vi "get Test by id.vi"(8 "error in (no error)":errorcluster, 10 "id":i32, 11 "Norm in":refnum<class "Norm.lvclass">) -> (0 "error out":errorcluster, 2 "Test.lvclass":refnum<class "Test.lvclass">, 3 "Norm out":refnum<class "Norm.lvclass">)   [LabVIEW 2013, in "DatenKlassen.lvlib" / "Norm.lvclass"]
uses:
  Norm.lvclass
  Test/Test.lvclass
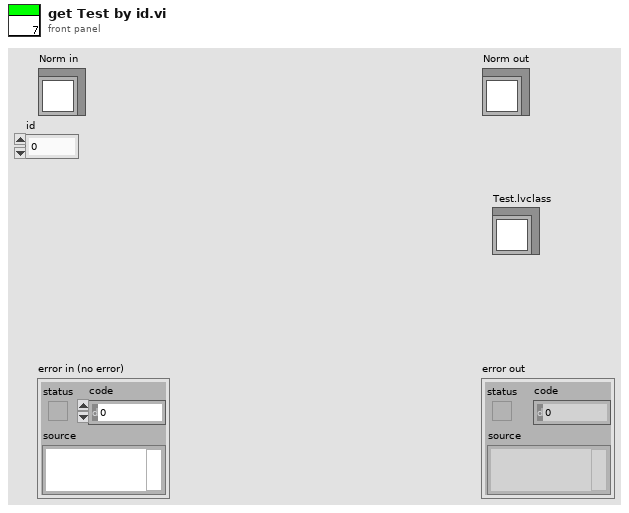
[diagram p1: front panel]
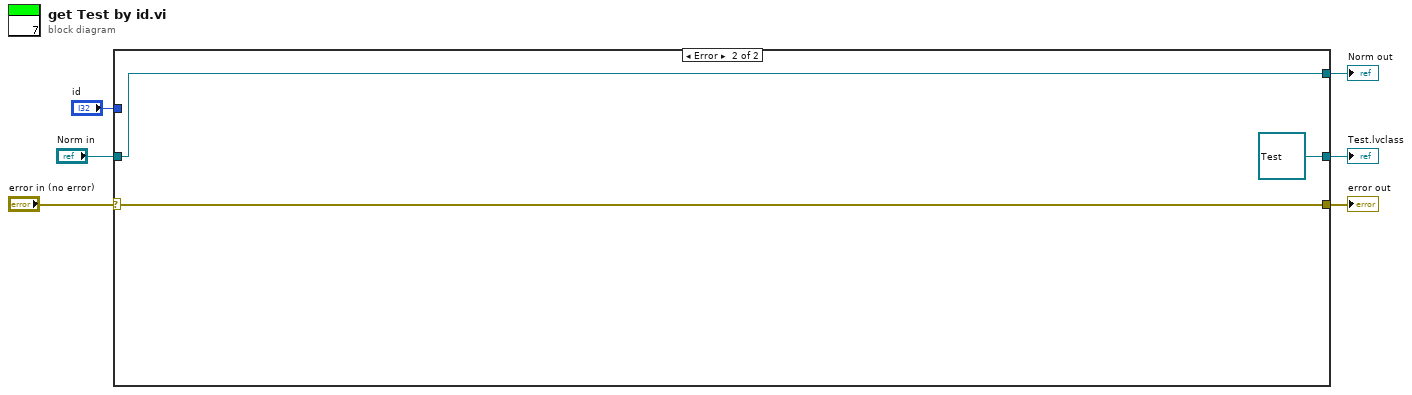
[diagram p0: block diagram]
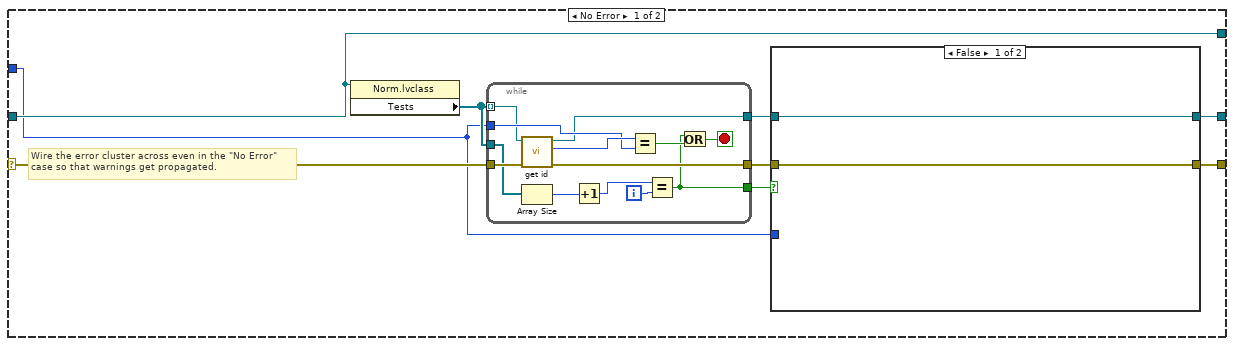
[diagram p2: hidden frame]
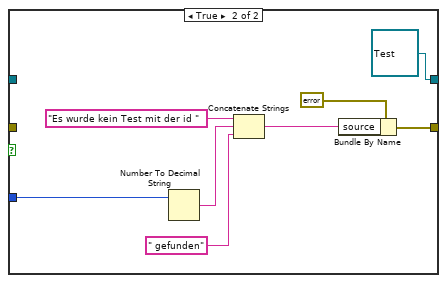
[diagram p3: hidden frame]
diagram:
  n1 = case shown="Error" "error in (no error)" {
    selector: "error in (no error)" -> [w14 w39]
    tunnel: [w9 w39] -> w5
    tunnel: [w15 w41] -> w3
    tunnel: "Norm in" -> [w15 w41]
    tunnel: "id" -> [w10 _]
    tunnel: [w8 refnum<class "Test.lvclass"> refnum ("Test out")] -> w1
    frame No Error {
      # "Wire the error cluster across even in the \"No Error\"\ncase so that warnings get propagated."
      n2 = property class="Norm.lvclass"(reference=w15) -> ("Tests"=w13:refnum<class "Test.lvclass">[])  [unwired: 1 in, 2 out]
      n3 = while {
        tunnel: w13 -> [w34] mode=indexing
        tunnel: w14 -> [w38]
        tunnel: w10 -> [w36]
        tunnel: [w35] -> w11
        tunnel: w13 -> [w33]
        tunnel: [w27] -> w12
        tunnel: [w26] -> w7
        i -> [w32]
        stop <- w30 stop-if-true
        n4 = call-dynamic "get id.vi"("error in (no error)"=w38, "Test in"=w34) -> ("error out"=w35:errorcluster, "id"=w37:u32, "Test out"=w26:refnum<class "Test.lvclass">)  [unwired: 7 in]
        n5 = Array Size(array=w33) -> (size(s)=w29:i32)
        n6 = Increment(x=w29) -> (x+1=w28:i32)
        n7 = Equal?(x=w37, y=w36) -> (x = y?=w31:bool)
        n8 = Equal?(x=w28, y=w32) -> (x = y?=w27:bool)
        n9 = Or(x=w27, y=w31) -> (x .or. y?=w30:bool)
      }
      n10 = case shown="False" w12 {
        tunnel: w11 -> [w16 _]
        tunnel: w10 -> [_ w23]
        tunnel: [w16 w20] -> w9
        tunnel: [w17 refnum<class "Test.lvclass"> refnum ("Test out")] -> w8
        tunnel: w7 -> [w17 _]
        frame False {
        }
        frame True {
          n11 = Number To Decimal String(number=w23) -> (decimal integer string=w22:string)  [unwired: 1 in]
          n12 = Concatenate Strings("Es wurde kein Test mit der id " ("source"), w22, " gefunden" ("string")) -> (w19:string)
          n13 = Bundle By Name(cluster=errorcluster {"status"=TRUE, "code"=9999, "source"="Es wurde kein Test mit der id "} ("error constant"), "source"=w19) -> (w20:errorcluster)
        }
      }
    }
    frame Error {
    }
  }
  "error out" <- w5
  "Norm out" <- w3
  "Test.lvclass" <- w1
